vi "WriteTree.vi"(8 "error in":errorcluster, 11 "SequenceRepo in":refnum<class "SequenceRepo.lvclass">) -> (0 "error out":errorcluster, 2 "root":T1, 3 "repository out":refnum<class "NISE_CEF_Repository.lvclass">)   [LabVIEW 2015, in "SequenceRepo.lvclass"]
doc: "Copyright 2017 National Instruments Corporation\n\nLicensed under the Apache License, Version 2.0 (the \"License\"); you may not use this file except in compliance with the License. You may obtain a copy of the License at http://www.apache.org/licenses/LICENSE-2.0\nUnless required by applicable law or agreed to in writing, software distributed under the License is distributed on an \"AS IS\" BASIS, WITHOUT WARRANTIES OR CONDITIONS OF ANY KIND, either express or implied. See the License for the specific language governing permissions and limitations under the License."
uses:
  SequenceRepo.lvclass
  <vilib>/NI/Configuration Framework/Repository/NISE_CEF_Repository.lvclass
  <vilib>/NI/Configuration Framework/Node/NodeRef.ctl
  <vilib>/NI/Configuration Framework/Node/NISE_CEF_Node.lvclass
  SequenceNode/SequenceNode.lvclass
  <vilib>/NI/Configuration Framework/hierarchy repo/NISE_CEF_HierarchyRepo.lvclass
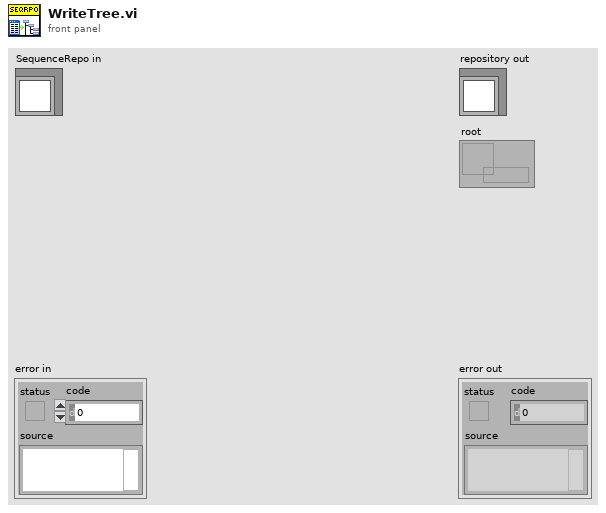
[diagram p1: front panel]
types:
  T1 = typedef "NISE_CEF_Node.lvclass/NodeRef.ctl" = refnum<data-value>
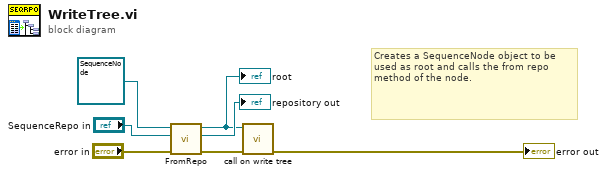
[diagram p0: block diagram]
diagram:
  # "Creates a SequenceNode object to be used as root and calls the from repo method of the node."
  n1 = call-dynamic "FromRepo.vi"("error in"="error in", "repository in"="SequenceRepo in", "SequenceNode in"=refnum<class "SequenceNode.lvclass"> refnum ("cRIO.lvclass")) -> ("error out"=w3:errorcluster, "repository out"=→"repository out":refnum<class "NISE_CEF_Repository.lvclass">, "node"=w2:T1)  [unwired: 6 in]
  "root" <- w2
  n2 = call <vilib>:"call on write tree.vi"("error in"=w3, "root"=w2) -> ("error out"=→"error out":errorcluster)  [unwired: 9 in]
